vi "debugging probe.vi"(6 "Data Type":enum16{"Data Only", "Type Only", "Data & Type"}(ring), 7 "Export to (Dialog)":T1(ring), 8 "error in":errorcluster, 11 "Any Data":variant) -> (0 "error out":errorcluster, 3 "text":string)   [LabVIEW 2020, in "Reusable Library.lvlib"]
uses:
  Reusable Library.lvlib
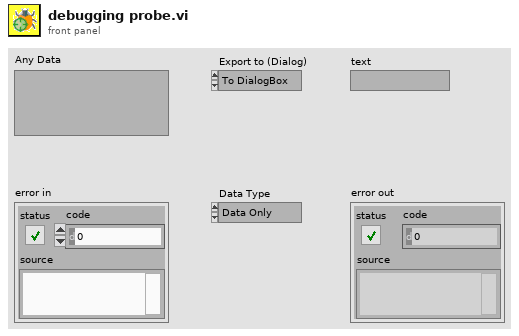
[diagram p1: front panel]
types:
  T1 = enum16{"To DialogBox", "To ClipBoard", "Serialize"}
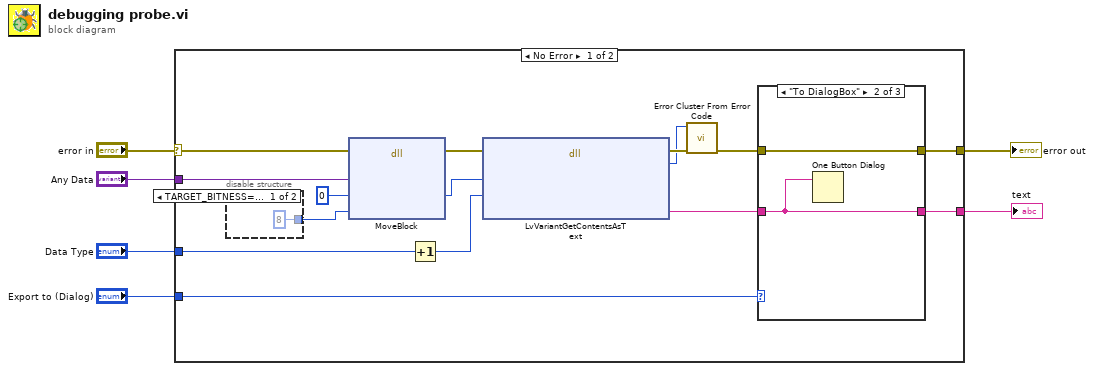
[diagram p0: block diagram]
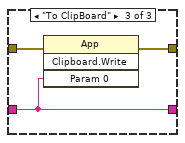
[diagram p3: hidden frame]
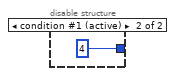
[diagram p4: hidden frame]
diagram:
  n1 = case shown="No Error" "error in" {
    selector: "error in" -> [w15 w31]
    tunnel: "Any Data" -> [w14 _]
    tunnel: "Data Type" -> [w13 _]
    tunnel: [w10 w31] -> w3
    tunnel: "Export to (Dialog)" -> [w9 _]
    tunnel: [w8 _] -> w1
    frame No Error {
      n2 = disable-structure shown="TARGET_BITNESS==64" {
        disable-tunnel: [u64 8 ("size") u64 4 ("size")] -> w17
        frame condition #0 {
        }
        frame condition #1 (active) {
        }
      }
      n3 = dll-call lib="LabVIEW" fn="MoveBlock"(error in=w15, "src"=w14, "tgt"=u64 0, "size"=w17) -> (error out=w19:errorcluster, "tgt"=w18:u64)  [unwired: 5 in, 1 out]
      n4 = Increment(x=w13) -> (x+1=w12:enum16{"Data Only", "Type Only", "Data & Type"})
      n5 = dll-call lib="LabVIEW" fn="LvVariantGetContentsAsText"(error in=w19, "variant"=w18, "displayStyle"=w12) -> (error out=w21:errorcluster, "err"=w20:i32, "string"=w7:string)  [unwired: 5 in, 1 out]
      n6 = call <vilib>:"Error Cluster From Error Code.vi"("error in (no error)"=w21, "error code (0)"=w20) -> ("error out"=w11:errorcluster)  [unwired: 7 in]
      n7 = case shown="\"To DialogBox\"" w9 {
        tunnel: w11 -> [w23 w25 w28]
        tunnel: [w23 w25 w27] -> w10
        tunnel: [w22 w24 w26] -> w8
        tunnel: w7 -> [w22 w24 w26]
        frame "Serialize", Default {
        }
        frame "To DialogBox" {
          n8 = One Button Dialog(message=w24) -> ()  [unwired: 1 in, 1 out]
        }
        frame "To ClipBoard" {
          n9 = invoke class="App" method="Clipboard.Write"(error in=w28, "Param 0"=w26) -> (error out=w27:errorcluster)  [unwired: 2 in, 3 out]
        }
      }
    }
    frame Error {
    }
  }
  "error out" <- w3
  "text" <- w1
